vi "Teff_Calc_Single.vi"(9 "Bed Temp":dbl, 10 "TRF":dbl) -> (2 "Teff":dbl)   [LabVIEW 2014]
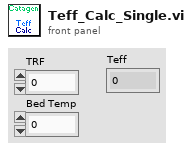
[diagram p1: front panel]
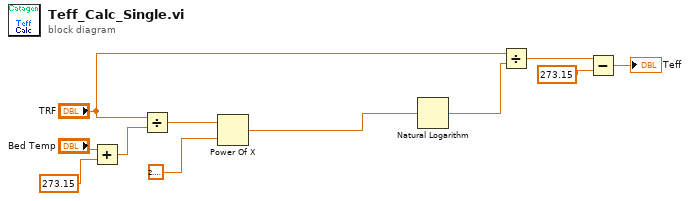
[diagram p0: block diagram]
diagram:
  n1 = Add(x="Bed Temp", y=273.15) -> (x+y=w2:dbl)
  n2 = Divide(x="TRF", y=w2) -> (x/y=w11:dbl)
  n3 = Power Of X(1:2.718281828459045, 2:w11) -> (0:w4:dbl)
  n4 = Natural Logarithm(1:w4) -> (0:w9:dbl)
  n5 = Divide(x="TRF", y=w9) -> (x/y=w6:dbl)
  n6 = Subtract(x=w6, y=273.15) -> (x-y=→"Teff":dbl)
